vi "Obtain Message Queue.vi"(8 "entrée d'erreur (pas d'erreur)":errorcluster) -> (0 "sortie d'erreur":errorcluster, 3 "File d'attente de messages":refnum<queue>)   [LabVIEW 2016, in "Message Queue.lvlib"]
doc: "Créer une file d'attente avec le type de données du cluster Message."
uses:
  Message Queue.lvlib
  Message Cluster.ctl
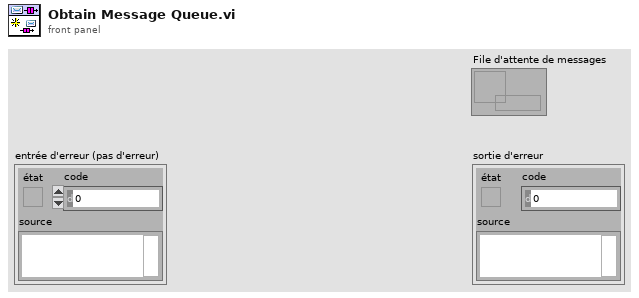
[diagram p1: front panel]
types:
  T1 = typedef "Message Queue.lvlib/Message Cluster.ctl" = cluster{"Message":string, "Données de message":variant}
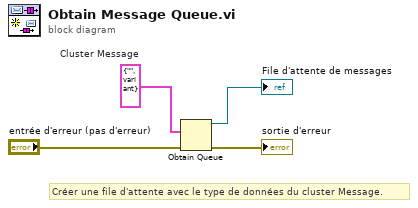
[diagram p0: block diagram]
diagram:
  w4 = T1 {"Message"="", "Données de message"=variant}  # Cluster Message
  # "Créer une file d'attente avec le type de données du cluster Message."
  n1 = Obtain Queue(element data type=w4, error in (no error)="entrée d'erreur (pas d'erreur)") -> (queue out=→"File d'attente de messages":refnum<queue>, error out=→"sortie d'erreur":errorcluster)  [unwired: 3 in, 1 out]
